vi "roverView.vi"() -> ()   [LabVIEW 2023]
uses:
  globalVariables.vi
panel:
  in  "Simulation stop":bool
  out "Back right wheel":dbl(graph)
  out "Back left wheel":dbl(graph)
  out "Front right wheel":dbl(graph)
  out "Front left wheel":dbl(graph)
  out "Velocity of the rover's left-side wheels":dbl(graph)
  out "Rover wheel velocity on the right side":string
  out "Scientific notation":dbl
  out "Scientific notation":dbl
  out "Rover wheel velocity on the left side":string
  out "Velocity of the rover's right-side wheels":dbl(graph)
  out "standard output 2":string
  out "ASCII Char 3":i16
  out "Character 2":string
  out "System user":string
  out "Simulation time":dbl
  out "Movement log":string
  out "Keys pressed log":string
  out "Key pressed":string
  out "Detected movement indicator":string
  out "ASCII Char 2":i16
  out "ASCII Char":i16
  out "Character":string
  out "standard output":string
  # "Rover control"
  # "Logs"
  # "Wheel movement charts"
  # "Movement data"
  # "Velocity charts"
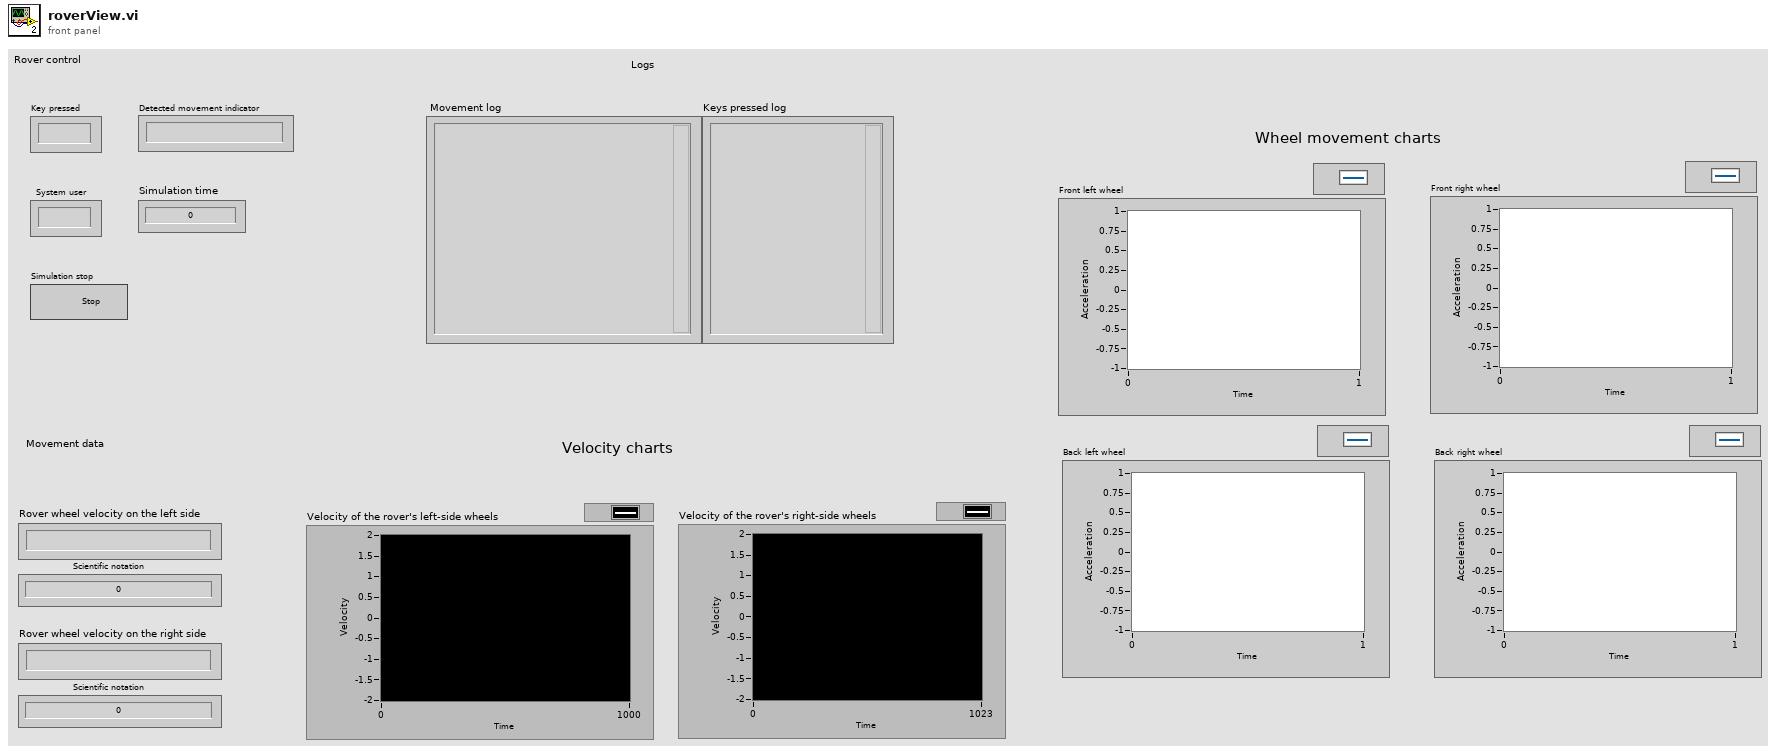
[diagram p1: front panel]
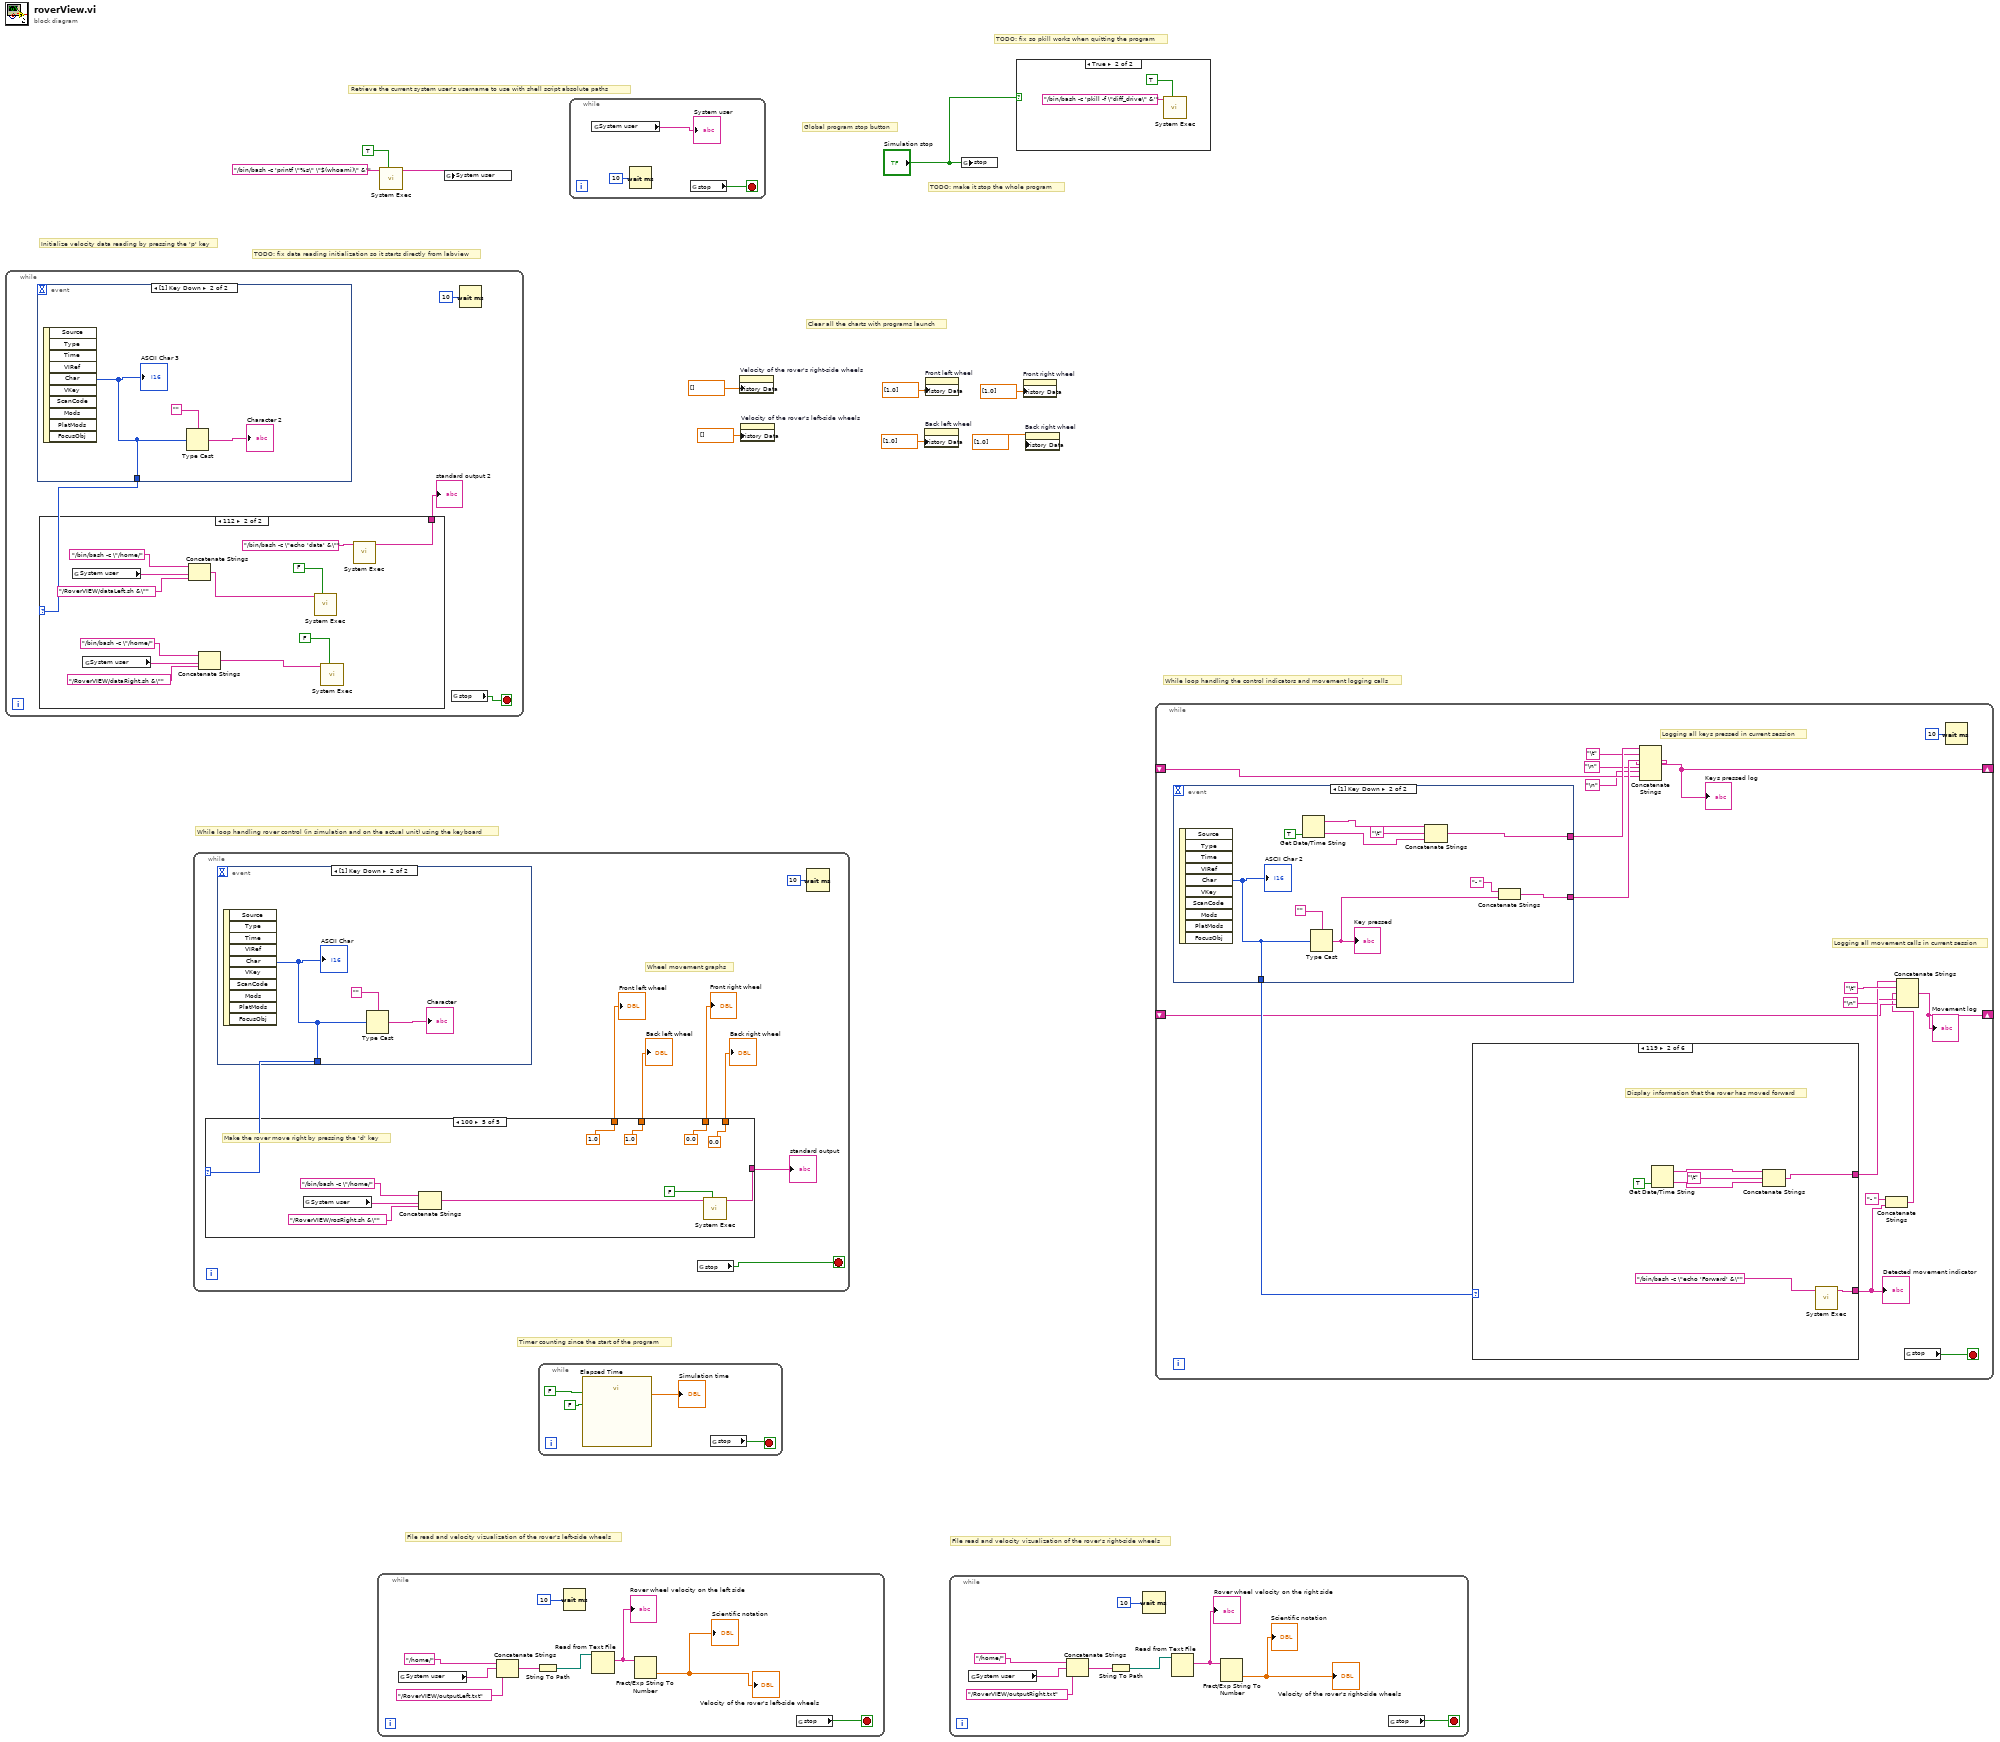
[diagram p0: block diagram]
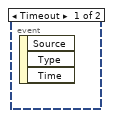
[diagram p3: hidden frame]
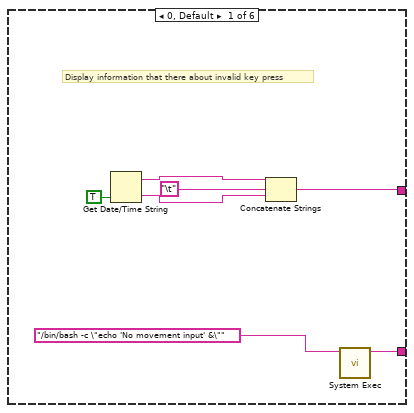
[diagram p5: hidden frame]
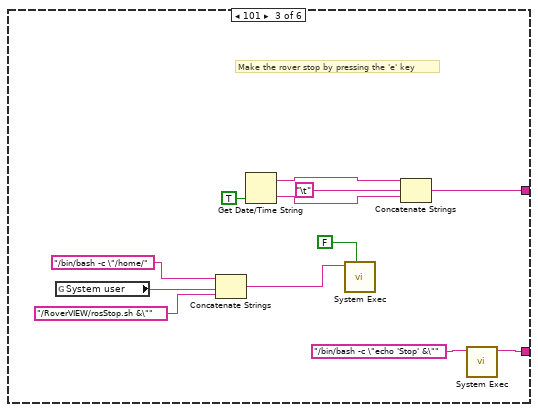
[diagram p6: hidden frame]
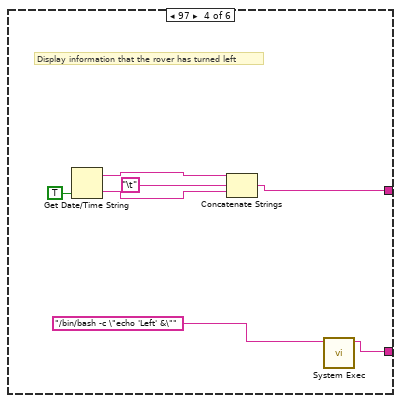
[diagram p7: hidden frame]
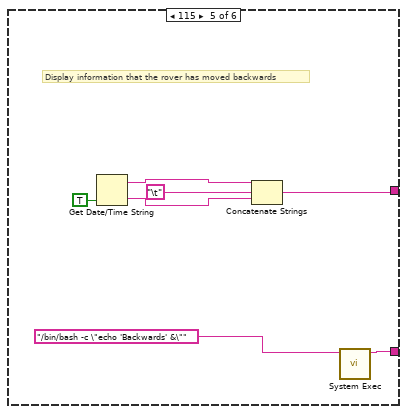
[diagram p8: hidden frame]
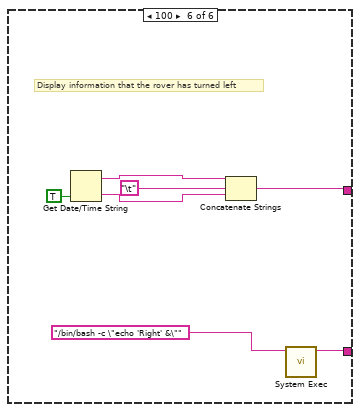
[diagram p9: hidden frame]
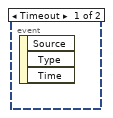
[diagram p10: hidden frame]
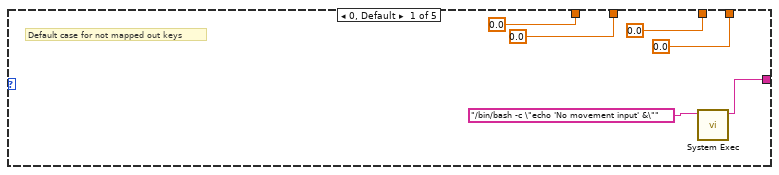
[diagram p11: hidden frame]
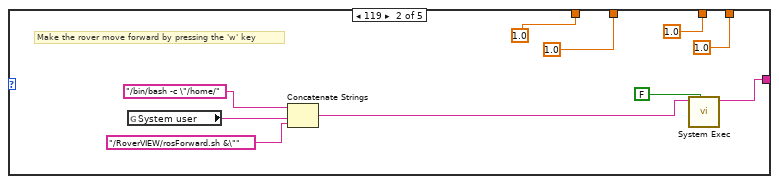
[diagram p12: hidden frame]
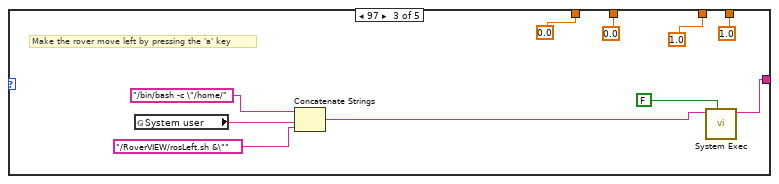
[diagram p13: hidden frame]
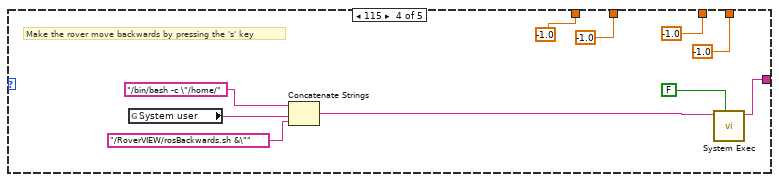
[diagram p14: hidden frame]
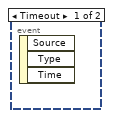
[diagram p15: hidden frame]
diagram:
  # "TODO: fix so pkill works when quitting the program"
  # "Clear all the charts with programs launch"
  # "TODO: fix data reading initialization so it starts directly from labview"
  # "TODO: make it stop the whole program"
  # "Global program stop button"
  # "Initialize velocity data reading by pressing the 'p' key"
  # "File read and velocity vizualization of the rover's right-side wheels"
  # "File read and velocity vizualization of the rover's left-side wheels"
  # "Timer counting since the start of the program"
  # "Retrieve the current system user's username to use with shell script absolute paths"
  # "While loop handling the control indicators and movement logging calls"
  # "While loop handling rover control (in simulation and on the actual unit) using the keyboard"
  n1 = while {
    stop <- w11 stop-if-true
    n2 = event shown="[1] Key Down" {
      selector: _ -> [_ _]
      dyn-events: _ -> [_ _]
      timeout: _ -> [_ _]
      tunnel: [_ w15] -> w14
      event Timeout {
        n3 = event-data() -> ()  [unwired: 1 in, 3 out]
      }
      event Key Down {
        n4 = event-data() -> ("Char"=w15:i16)  [unwired: 1 in, 9 out]
        "ASCII Char 3" <- w15
        n5 = Type Cast(type="", x=w15) -> (*(type *) &x=→"Character 2":string)
      }
    }
    n6 = case shown="112" w14 {
      tunnel: [_ w26] -> w13
      frame 0, Default {
      }
      frame 112 {
        n7 = global read "globalVariables.vi" "System user"() -> (w20:string)
        n8 = global read "globalVariables.vi" "System user"() -> (w24:string)
        n9 = Concatenate Strings("/bin/bash -c \"/home/", w20, "/RoverVIEW/dataLeft.sh &\"") -> (w18:string)
        n10 = Concatenate Strings("/bin/bash -c \"/home/", w24, "/RoverVIEW/dataRight.sh &\"") -> (w22:string)
        n11 = call <vilib>:"System Exec.vi"("wait until completion? (T)"=FALSE, "command line"=w18) -> ()  [unwired: 6 in, 4 out]
        n12 = call <vilib>:"System Exec.vi"("wait until completion? (T)"=FALSE, "command line"=w22) -> ()  [unwired: 6 in, 4 out]
        n13 = call <vilib>:"System Exec.vi"("command line"="/bin/bash -c \"echo 'data' &\"") -> ("standard output"=w26:string)  [unwired: 7 in, 3 out]
      }
    }
    "standard output 2" <- w13
    n14 = global read "globalVariables.vi" "stop"() -> (w11:bool)
    n15 = Wait (ms)(milliseconds to wait=u32 10) -> ()  [unwired: 1 out]
  }
  n16 = while {
    stop <- w30 stop-if-true
    # "Wheel movement graphs"
    n17 = event shown="[1] Key Down" {
      selector: _ -> [_ _]
      dyn-events: _ -> [_ _]
      timeout: _ -> [_ _]
      tunnel: [_ w84] -> w37
      event Timeout {
        n18 = event-data() -> ()  [unwired: 1 in, 3 out]
      }
      event Key Down {
        n19 = event-data() -> ("Char"=w84:i16)  [unwired: 1 in, 9 out]
        "ASCII Char" <- w84
        n20 = Type Cast(type="", x=w84) -> (*(type *) &x=→"Character":string)
      }
    }
    n21 = case shown="100" w37 {
      tunnel: [w42 w53 w63 w73 w83] -> w36
      tunnel: [0.0 1.0 0.0 -1.0 1.0] -> w31
      tunnel: [0.0 1.0 0.0 -1.0 1.0] -> w34
      tunnel: [0.0 1.0 1.0 -1.0 0.0] -> w33
      tunnel: [0.0 1.0 1.0 -1.0 0.0] -> w32
      frame 0, Default {
        # "Default case for not mapped out keys"
        n22 = call <vilib>:"System Exec.vi"("command line"="/bin/bash -c \"echo 'No movement input' &\"") -> ("standard output"=w42:string)  [unwired: 7 in, 3 out]
      }
      frame 119 {
        # "Make the rover move forward by pressing the 'w' key"
        n23 = global read "globalVariables.vi" "System user"() -> (w50:string)
        n24 = Concatenate Strings("/bin/bash -c \"/home/", w50, "/RoverVIEW/rosForward.sh &\"") -> (w48:string)
        n25 = call <vilib>:"System Exec.vi"("wait until completion? (T)"=FALSE, "command line"=w48) -> ("standard output"=w53:string)  [unwired: 6 in, 3 out]
      }
      frame 97 {
        # "Make the rover move left by pressing the 'a' key"
        n26 = global read "globalVariables.vi" "System user"() -> (w60:string)
        n27 = Concatenate Strings("/bin/bash -c \"/home/", w60, "/RoverVIEW/rosLeft.sh &\"") -> (w58:string)
        n28 = call <vilib>:"System Exec.vi"("wait until completion? (T)"=FALSE, "command line"=w58) -> ("standard output"=w63:string)  [unwired: 6 in, 3 out]
      }
      frame 115 {
        # "Make the rover move backwards by pressing the 's' key"
        n29 = global read "globalVariables.vi" "System user"() -> (w70:string)
        n30 = Concatenate Strings("/bin/bash -c \"/home/", w70, "/RoverVIEW/rosBackwards.sh &\"") -> (w68:string)
        n31 = call <vilib>:"System Exec.vi"("wait until completion? (T)"=FALSE, "command line"=w68) -> ("standard output"=w73:string)  [unwired: 6 in, 3 out]
      }
      frame 100 {
        # "Make the rover move right by pressing the 'd' key"
        n32 = global read "globalVariables.vi" "System user"() -> (w80:string)
        n33 = Concatenate Strings("/bin/bash -c \"/home/", w80, "/RoverVIEW/rosRight.sh &\"") -> (w78:string)
        n34 = call <vilib>:"System Exec.vi"("wait until completion? (T)"=FALSE, "command line"=w78) -> ("standard output"=w83:string)  [unwired: 6 in, 3 out]
      }
    }
    "standard output" <- w36
    "Front left wheel" <- w31
    "Front right wheel" <- w33
    "Back left wheel" <- w34
    "Back right wheel" <- w32
    n35 = global read "globalVariables.vi" "stop"() -> (w30:bool)
    n36 = Wait (ms)(milliseconds to wait=u32 10) -> ()  [unwired: 1 out]
  }
  n37 = while {
    stop <- w87 stop-if-true
    n38 = global read "globalVariables.vi" "System user"() -> (w92:string)
    n39 = Concatenate Strings("/home/", w92, "/RoverVIEW/outputLeft.txt") -> (w90:string)
    n40 = String To Path(string=w90) -> (path=w94:path)
    n41 = Wait (ms)(milliseconds to wait=u32 10) -> ()  [unwired: 1 out]
    n42 = Read from Text File(file (use dialog)=w94) -> (text=w89:string)  [unwired: 3 in, 3 out]
    "Rover wheel velocity on the left side" <- w89
    n43 = Fract/Exp String To Number(string=w89) -> (number=→"Scientific notation" →"Velocity of the rover's left-side wheels":dbl)  [unwired: 3 in, 1 out]
    n44 = global read "globalVariables.vi" "stop"() -> (w87:bool)
  }
  n45 = call <vilib>:"System Exec.vi"("wait until completion? (T)"=TRUE, "command line"="/bin/bash -c 'printf \"%s\" \"$(whoami)\" &'") -> ("standard output"=w10:string)  [unwired: 6 in, 3 out]
  n46 = global write "globalVariables.vi" "System user"(w10) -> ()
  n47 = while {
    stop <- w96 stop-if-true
    n48 = call "Elapsed Time"("Reset"=FALSE, "Auto Reset"=FALSE) -> ("Elapsed Time (s)"=→"Simulation time":dbl)  [unwired: 10 in, 7 out]
    n49 = global read "globalVariables.vi" "stop"() -> (w96:bool)
  }
  n50 = while {
    stop <- w100 stop-if-true
    n51 = global read "globalVariables.vi" "System user"() -> (→"System user":string)
    n52 = Wait (ms)(milliseconds to wait=u32 10) -> ()  [unwired: 1 out]
    n53 = global read "globalVariables.vi" "stop"() -> (w100:bool)
  }
  n54 = property on="Velocity of the rover's right-side wheels" class="WFChart (strict)"("History Data"=dbl[] []) -> ()  [unwired: 2 in, 2 out]
  n55 = property on="Velocity of the rover's left-side wheels" class="WFChart (strict)"("History Data"=dbl[] []) -> ()  [unwired: 2 in, 2 out]
  n56 = property on="Back left wheel" class="WFChart (strict)"("History Data"=dbl[] [1.0]) -> ()  [unwired: 2 in, 2 out]
  n57 = property on="Front left wheel" class="WFChart (strict)"("History Data"=dbl[] [1.0]) -> ()  [unwired: 2 in, 2 out]
  n58 = while {
    stop <- w103 stop-if-true
    n59 = global read "globalVariables.vi" "System user"() -> (w109:string)
    n60 = Concatenate Strings("/home/", w109, "/RoverVIEW/outputRight.txt") -> (w107:string)
    n61 = String To Path(string=w107) -> (path=w106:path)
    n62 = Wait (ms)(milliseconds to wait=u32 10) -> ()  [unwired: 1 out]
    n63 = Read from Text File(file (use dialog)=w106) -> (text=w104:string)  [unwired: 3 in, 3 out]
    "Rover wheel velocity on the right side" <- w104
    n64 = Fract/Exp String To Number(string=w104) -> (number=→"Velocity of the rover's right-side wheels" →"Scientific notation":dbl)  [unwired: 3 in, 1 out]
    n65 = global read "globalVariables.vi" "stop"() -> (w103:bool)
  }
  n66 = global write "globalVariables.vi" "stop"("Simulation stop") -> ()
  n67 = case shown="True" "Simulation stop" {
    frame False {
    }
    frame True {
      n68 = call <vilib>:"System Exec.vi"("wait until completion? (T)"=TRUE, "command line"="/bin/bash -c 'pkill -f \"diff_drive\" &'") -> ()  [unwired: 6 in, 4 out]
    }
  }
  n69 = property on="Front right wheel" class="WFChart (strict)"("History Data"=dbl[] [1.0]) -> ()  [unwired: 2 in, 2 out]
  n70 = property on="Back right wheel" class="WFChart (strict)"("History Data"=dbl[] [1.0]) -> ()  [unwired: 2 in, 2 out]
  n71 = while {
    shift-right: [w125] -> _
    shift-left: _ -> [w116]
    shift-right: [w124] -> _
    shift-left: _ -> [w120]
    stop <- w114 stop-if-true
    # "Logging all movement calls in current session"
    # "Logging all keys pressed in current session"
    n72 = event shown="[1] Key Down" {
      selector: _ -> [_ _]
      dyn-events: _ -> [_ _]
      timeout: _ -> [_ _]
      tunnel: [_ w187] -> w131
      tunnel: [_ w183] -> w129
      tunnel: [_ w179] -> w128
      event Timeout {
        n73 = event-data() -> ()  [unwired: 1 in, 3 out]
      }
      event Key Down {
        n74 = event-data() -> ("Char"=w187:i16)  [unwired: 1 in, 9 out]
        "ASCII Char 2" <- w187
        n75 = Get Date/Time String(want seconds? (F)=TRUE) -> (date string=w185:string, time string=w184:string)  [unwired: 2 in]
        n76 = Type Cast(type="", x=w187) -> (*(type *) &x=w180:string)
        "Key pressed" <- w180
        n77 = Concatenate Strings(w185, "\t", w184) -> (w183:string)
        n78 = Concatenate Strings("- " ("string"), w180) -> (w179:string)
      }
    }
    n79 = case shown="119" w131 {
      tunnel: [w137 w144 w156 w163 w170 w177] -> w117
      tunnel: [w132 w139 w150 w158 w165 w172] -> w122
      frame 0, Default {
        # "Display information that there about invalid key press"
        n80 = Get Date/Time String(want seconds? (F)=TRUE) -> (date string=w133:string, time string=w134:string)  [unwired: 2 in]
        n81 = Concatenate Strings(w133, "\t", w134) -> (w132:string)
        n82 = call <vilib>:"System Exec.vi"("command line"="/bin/bash -c \"echo 'No movement input' &\"") -> ("standard output"=w137:string)  [unwired: 7 in, 3 out]
      }
      frame 119 {
        # "Display information that the rover has moved forward"
        n83 = Get Date/Time String(want seconds? (F)=TRUE) -> (date string=w140:string, time string=w141:string)  [unwired: 2 in]
        n84 = Concatenate Strings(w140, "\t", w141) -> (w139:string)
        n85 = call <vilib>:"System Exec.vi"("command line"="/bin/bash -c \"echo 'Forward' &\"") -> ("standard output"=w144:string)  [unwired: 7 in, 3 out]
      }
      frame 101 {
        # "Make the rover stop by pressing the 'e' key"
        n86 = global read "globalVariables.vi" "System user"() -> (w148:string)
        n87 = Concatenate Strings("/bin/bash -c \"/home/", w148, "/RoverVIEW/rosStop.sh &\"") -> (w146:string)
        n88 = Get Date/Time String(want seconds? (F)=TRUE) -> (date string=w151:string, time string=w152:string)  [unwired: 2 in]
        n89 = call <vilib>:"System Exec.vi"("wait until completion? (T)"=FALSE, "command line"=w146) -> ()  [unwired: 6 in, 4 out]
        n90 = Concatenate Strings(w151, "\t", w152) -> (w150:string)
        n91 = call <vilib>:"System Exec.vi"("command line"="/bin/bash -c \"echo 'Stop' &\"") -> ("standard output"=w156:string)  [unwired: 7 in, 3 out]
      }
      frame 97 {
        # "Display information that the rover has turned left"
        n92 = Get Date/Time String(want seconds? (F)=TRUE) -> (date string=w159:string, time string=w160:string)  [unwired: 2 in]
        n93 = Concatenate Strings(w159, "\t", w160) -> (w158:string)
        n94 = call <vilib>:"System Exec.vi"("command line"="/bin/bash -c \"echo 'Left' &\"") -> ("standard output"=w163:string)  [unwired: 7 in, 3 out]
      }
      frame 115 {
        # "Display information that the rover has moved backwards"
        n95 = Get Date/Time String(want seconds? (F)=TRUE) -> (date string=w166:string, time string=w167:string)  [unwired: 2 in]
        n96 = Concatenate Strings(w166, "\t", w167) -> (w165:string)
        n97 = call <vilib>:"System Exec.vi"("command line"="/bin/bash -c \"echo 'Backwards' &\"") -> ("standard output"=w170:string)  [unwired: 7 in, 3 out]
      }
      frame 100 {
        # "Display information that the rover has turned left"
        n98 = Get Date/Time String(want seconds? (F)=TRUE) -> (date string=w173:string, time string=w174:string)  [unwired: 2 in]
        n99 = Concatenate Strings(w173, "\t", w174) -> (w172:string)
        n100 = call <vilib>:"System Exec.vi"("command line"="/bin/bash -c \"echo 'Right' &\"") -> ("standard output"=w177:string)  [unwired: 7 in, 3 out]
      }
    }
    "Detected movement indicator" <- w117
    n101 = Concatenate Strings(w129, "\t", w128, "\n", "\n", w116) -> (w125:string)
    "Keys pressed log" <- w125
    n102 = Concatenate Strings("- " ("string"), w117) -> (w119:string)
    n103 = Concatenate Strings(w122, "\t", w119, "\n", w120) -> (w124:string)
    "Movement log" <- w124
    n104 = global read "globalVariables.vi" "stop"() -> (w114:bool)
    n105 = Wait (ms)(milliseconds to wait=u32 10) -> ()  [unwired: 1 out]
  }
